vi "Generate Joint Trajectory.vi"   [LabVIEW 2017, in "NI_Kinematics.lvlib"]
doc: "Generates joint angles, velocities, and accelerations along a smooth trajectory between two points in joint space. Wire data to the <B>intermediate points</B> input to determine the polymorphic instance to use or manually select the instance.\n\n<B>.m file:</B> jtraj"
uses:
  <vilib>/robotics/Kinematics/NI_Kinematics.lvlib
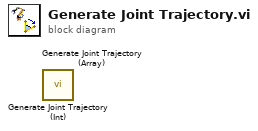
[diagram p0: block diagram]
diagram:
  n1 = call <vilib>:"Generate Joint Trajectory (Int).vi"() -> ()  [unwired: 8 in, 4 out]
  n2 = call <vilib>:"Generate Joint Trajectory (Array).vi"() -> ()  [unwired: 8 in, 4 out]
